vi "Rising Edge (Windowed).vi"(7 "Prior Lows":u8=10, 11 "Input":bool) -> (3 "Rising Edge?":bool)   [LabVIEW 2017]
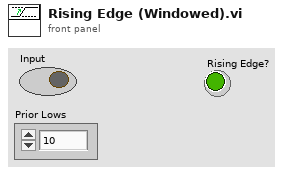
[diagram p1: front panel]
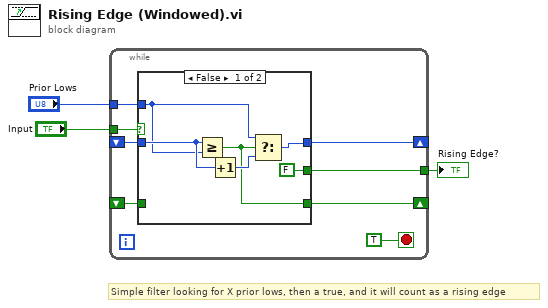
[diagram p0: block diagram]
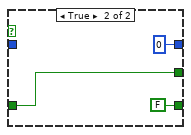
[diagram p2: hidden frame]
diagram:
  # "Simple filter looking for X prior lows, then a true, and it will count as a rising edge"
  n1 = while {
    tunnel: "Input" -> [w10]
    shift-right: [w8] -> _
    shift-left: _ -> [w9]
    shift-right: [w7] -> _
    shift-left: _ -> [w6]
    tunnel: [w5] -> w3
    tunnel: "Prior Lows" -> [w4]
    stop <- TRUE stop-if-true
    n2 = case shown="False" w10 {
      tunnel: w9 -> [w17 _]
      tunnel: [w15 u8 0 ("t")] -> w8
      tunnel: [w14 FALSE] -> w7
      tunnel: w6 -> [_ w18]
      tunnel: [FALSE w18] -> w5
      tunnel: w4 -> [w12 _]
      frame False {
        n3 = Greater Or Equal?(x=w17, y=w12) -> (x >= y?=w14:bool)
        n4 = Increment(x=w17) -> (x+1=w16:u8)
        n5 = Select(t=w12, s=w14, f=w16) -> (s? t:f=w15:u8)
      }
      frame True {
      }
    }
  }
  "Rising Edge?" <- w3
